vi "Compare_values_For_Cost_f()_Optimum-1.vi"(7 "[IN] Cost function":i8[](array[numeric]), 8 "[IN] Displ \ndifferences":dbl[](array[numeric]), 9 "[IN] Reverse or not":bool[](array[boolean]), 10 "[IN] Angles betwe\nen displacements":dbl[](array[numeric]), 11 "[IN] Array of displacements":dbl[](array[numeric])) -> (3 "[OUT] Cost function":i8[](array[numeric]))   [LabVIEW 2013]
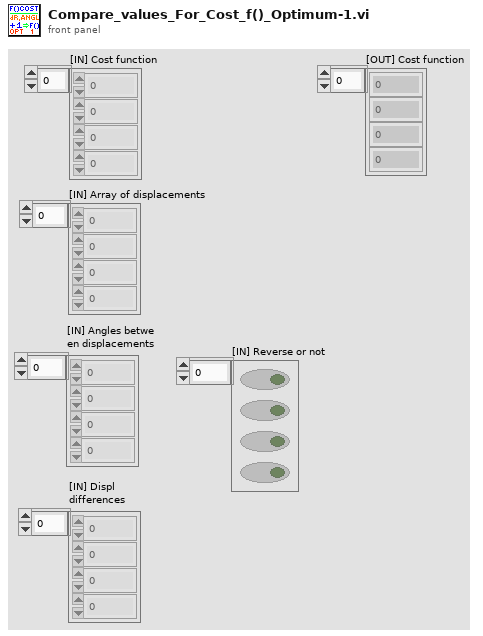
[diagram p1: front panel]
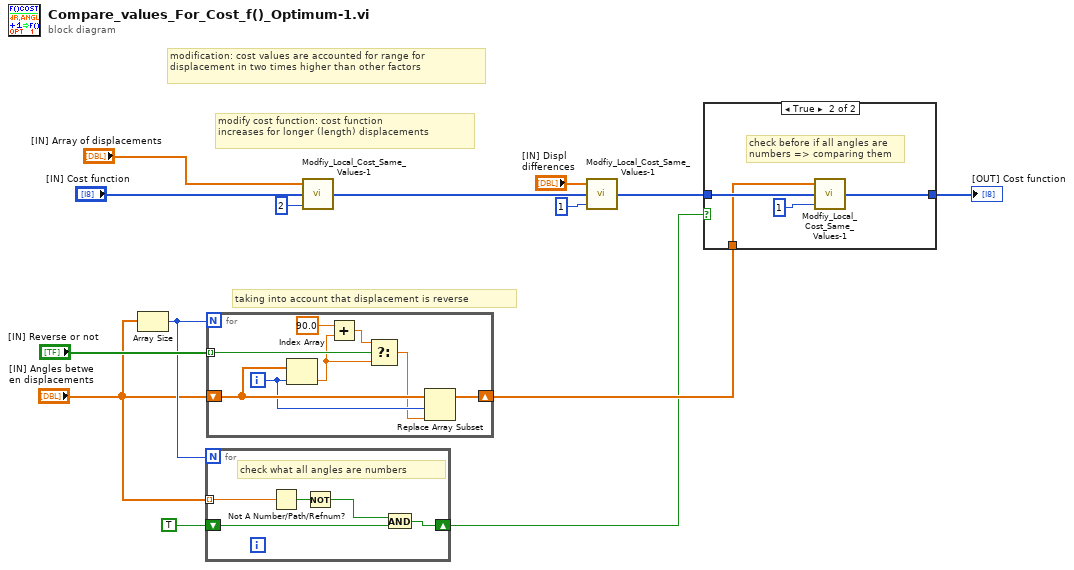
[diagram p0: block diagram]
diagram:
  # "modification: cost values are accounted for range for \ndisplacement in two times higher than other factors"
  # "taking into account that displacement is reverse"
  # "modify cost function: cost function \nincreases for longer (length) displacements"
  n1 = Array Size(array="[IN] Angles betwe\nen displacements") -> (size(s)=w12:i32)
  n2 = for {
    N: w12 -> [_]
    tunnel: "[IN] Angles betwe\nen displacements" -> [w18] mode=indexing
    shift-right: [w15] -> w10
    shift-left: TRUE -> [w19]
    # "check what all angles are numbers"
    n3 = Not A Number/Path/Refnum?(number/path/refnum=w18) -> (NaN/Path/Refnum?=w17:bool)
    n4 = Not(x=w17) -> (.not. x?=w16:bool)
    n5 = And(x=w16, y=w19) -> (x .and. y?=w15:bool)
  }
  n6 = for {
    N: w12 -> [_]
    shift-right: [w20] -> w13
    shift-left: "[IN] Angles betwe\nen displacements" -> [w26]
    tunnel: "[IN] Reverse or not" -> [w27] mode=indexing
    i -> [w22]
    n7 = Index Array(array=w26, index=w22) -> (element=w24:dbl)
    n8 = Add(x=90.0, y=w24) -> (x+y=w23:dbl)
    n9 = Select(t=w23, s=w27, f=w24) -> (s? t:f=w21:dbl)
    n10 = Replace Array Subset(array=w26, new element=w21, index=w22) -> (w20:dbl[])
  }
  n11 = call "Modfiy_Local_Cost_Same_Values-1.vi"("[IN] Cost Mutilplier"=i8 2 ("y"), "[IN] Cost Function"="[IN] Cost function", "[IN] Array of Compared Values"="[IN] Array of displacements") -> ("[OUT] Cost Function"=w4:i8[])  [unwired: 2 in]
  n12 = call "Modfiy_Local_Cost_Same_Values-1.vi"("[IN] Cost Mutilplier"=i8 1, "[IN] Cost Function"=w4, "[IN] Array of Compared Values"="[IN] Displ \ndifferences") -> ("[OUT] Cost Function"=w3:i8[])  [unwired: 2 in]
  n13 = case shown="True" w10 {
    tunnel: w13 -> [_ w31]
    tunnel: w3 -> [w28 w32]
    tunnel: [w28 w29] -> w9
    frame False {
    }
    frame True {
      # "check before if all angles are \nnumbers => comparing them"
      n14 = call "Modfiy_Local_Cost_Same_Values-1.vi"("[IN] Cost Mutilplier"=i8 1, "[IN] Cost Function"=w32, "[IN] Array of Compared Values"=w31) -> ("[OUT] Cost Function"=w29:i8[])  [unwired: 2 in]
    }
  }
  "[OUT] Cost function" <- w9
